vi "NI 9203_DOUBLETASK_AI.vi"(0 "MODULE NAME":string="CDR_AI", 1 "MODULE NAME 2":string="CDR_AI", 2 "sample mode":i32(ring)=10178 items=["Finite Samples"=10178, "Continuous Samples"=10123, "Hardware Timed Single Point"=12522], 3 "double task?":bool, 4 "rate":dbl=1000.0 format="%0.2f", 5 "error in":errorcluster) -> (14 "task out":refnum<k21>, 19 "error out":errorcluster)   [LabVIEW 2016]
uses:
  <vilib>/DAQmx/configure/timing.llb/DAQmx Timing (Sample Clock).vi
  <vilib>/DAQmx/create/channels.llb/DAQmx Create Channel (AI-Current-Basic).vi
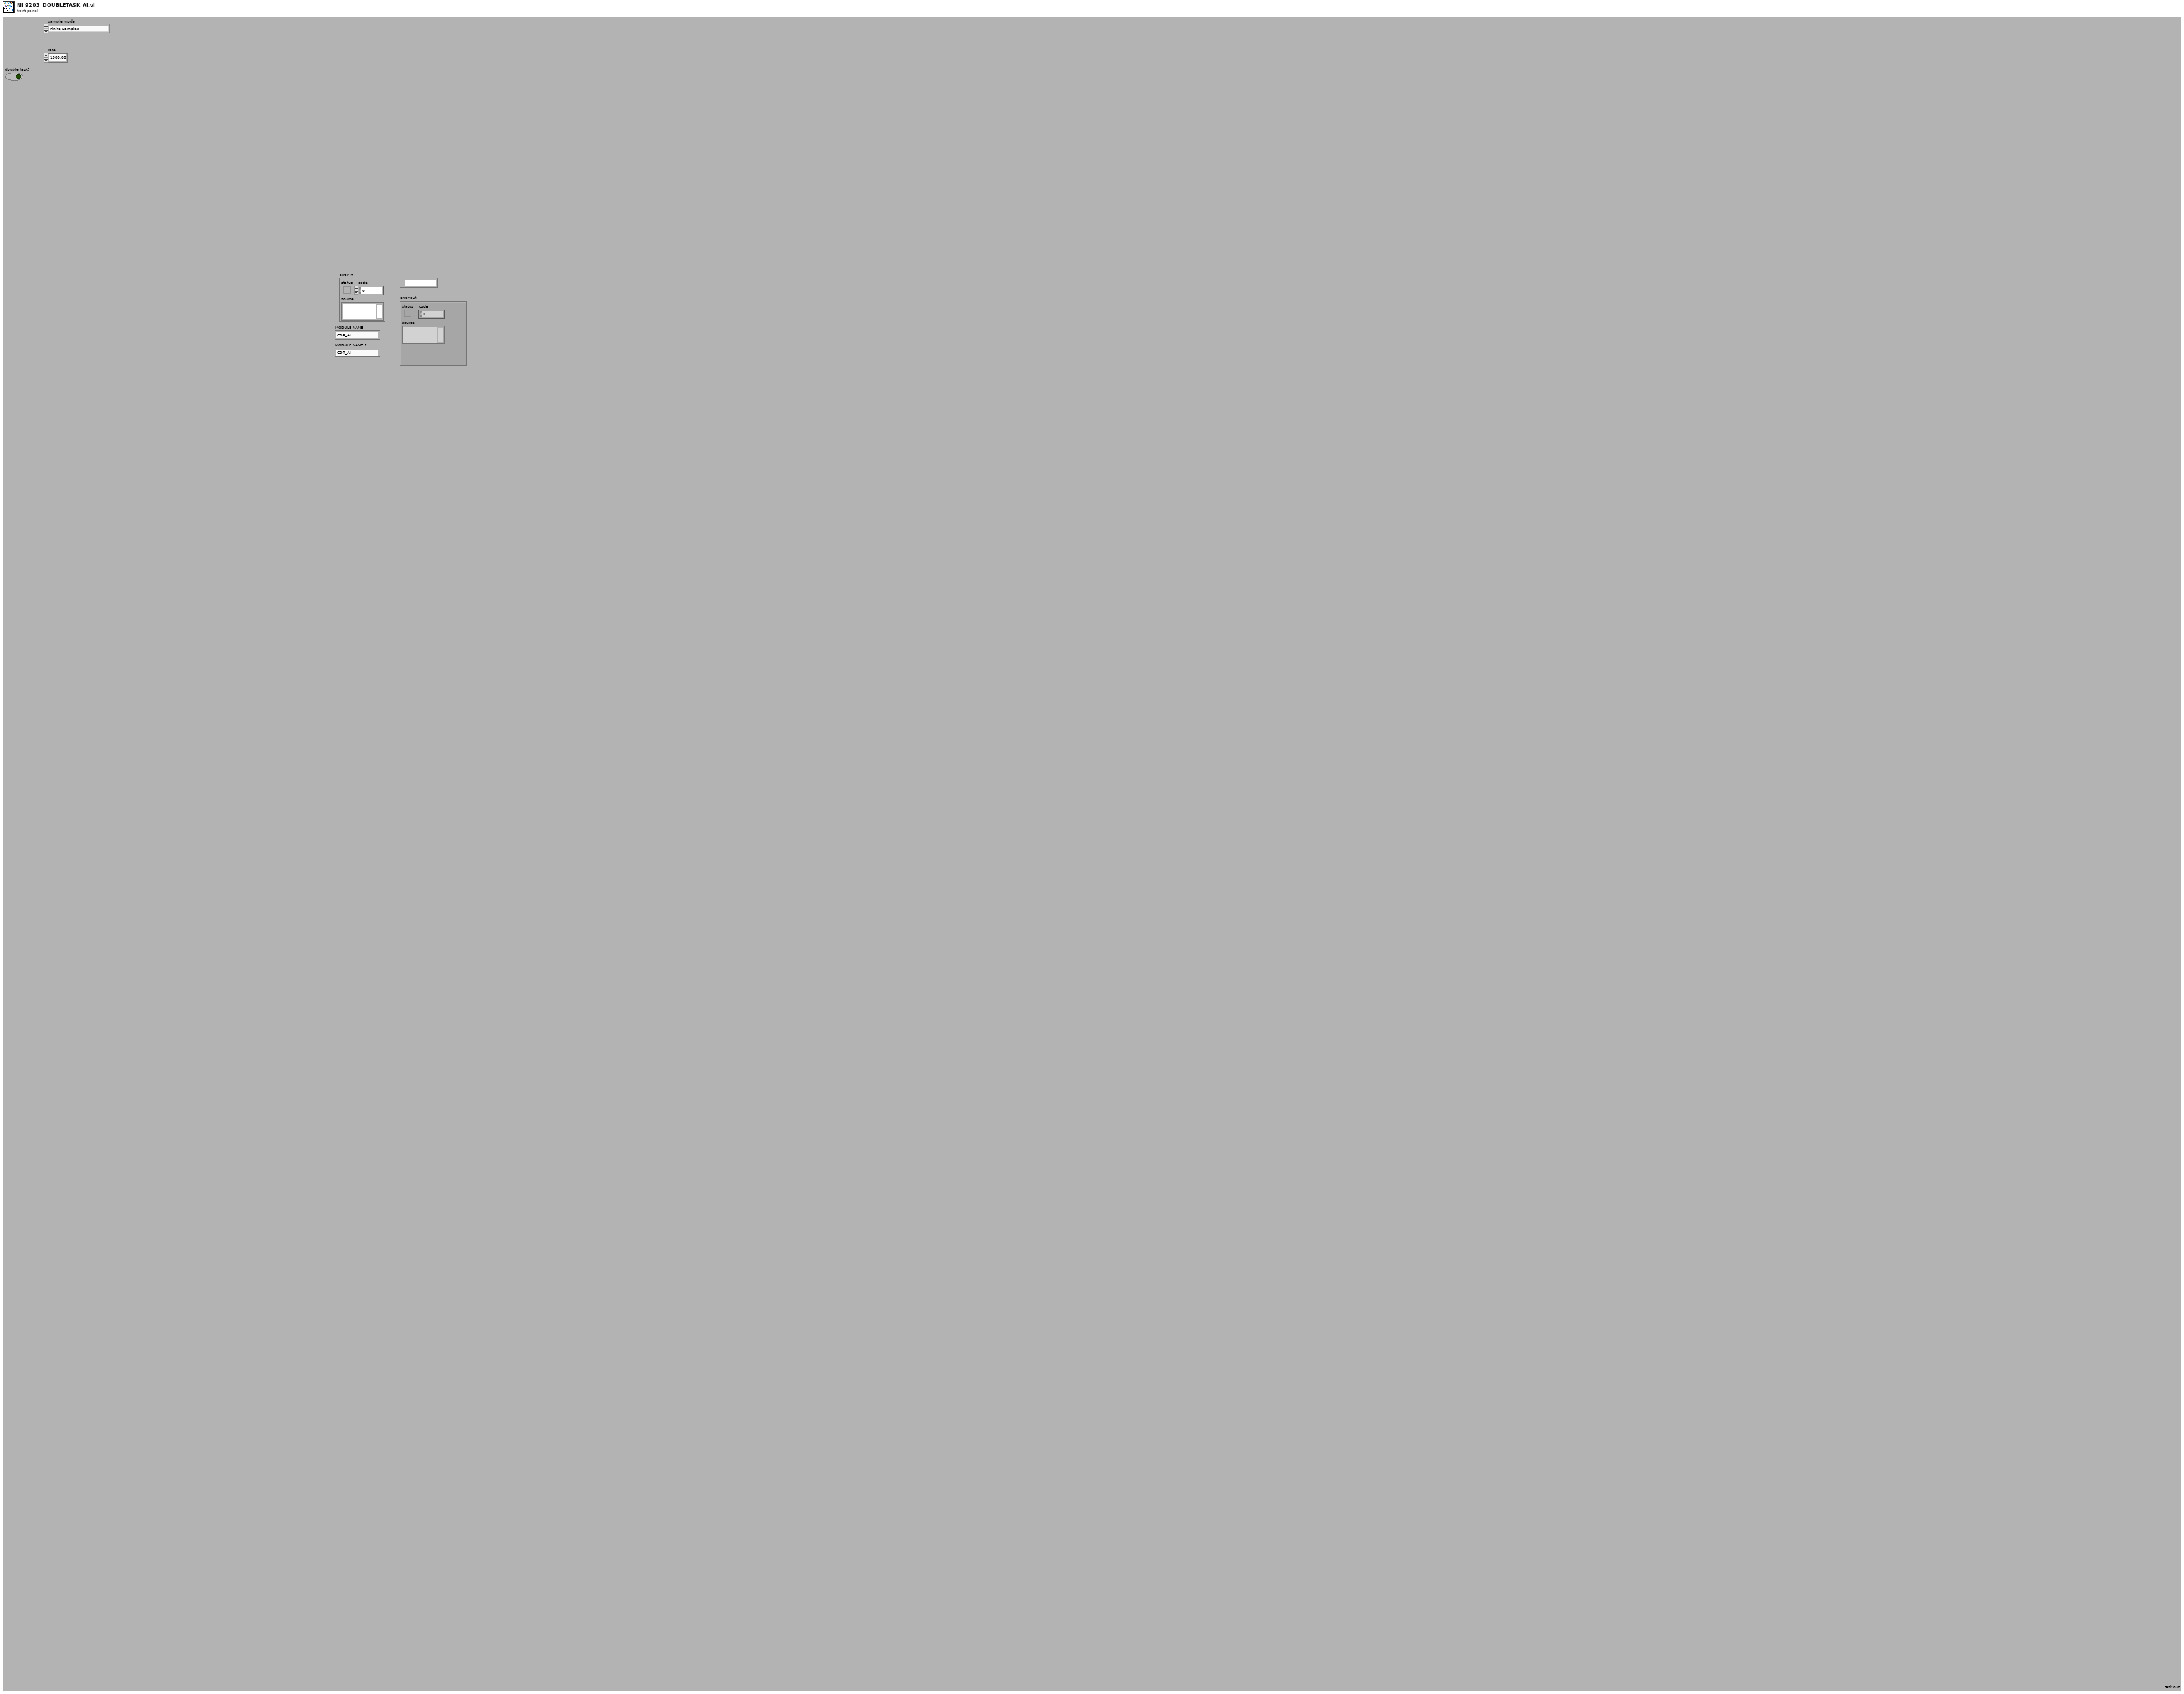
[diagram p1: front panel]
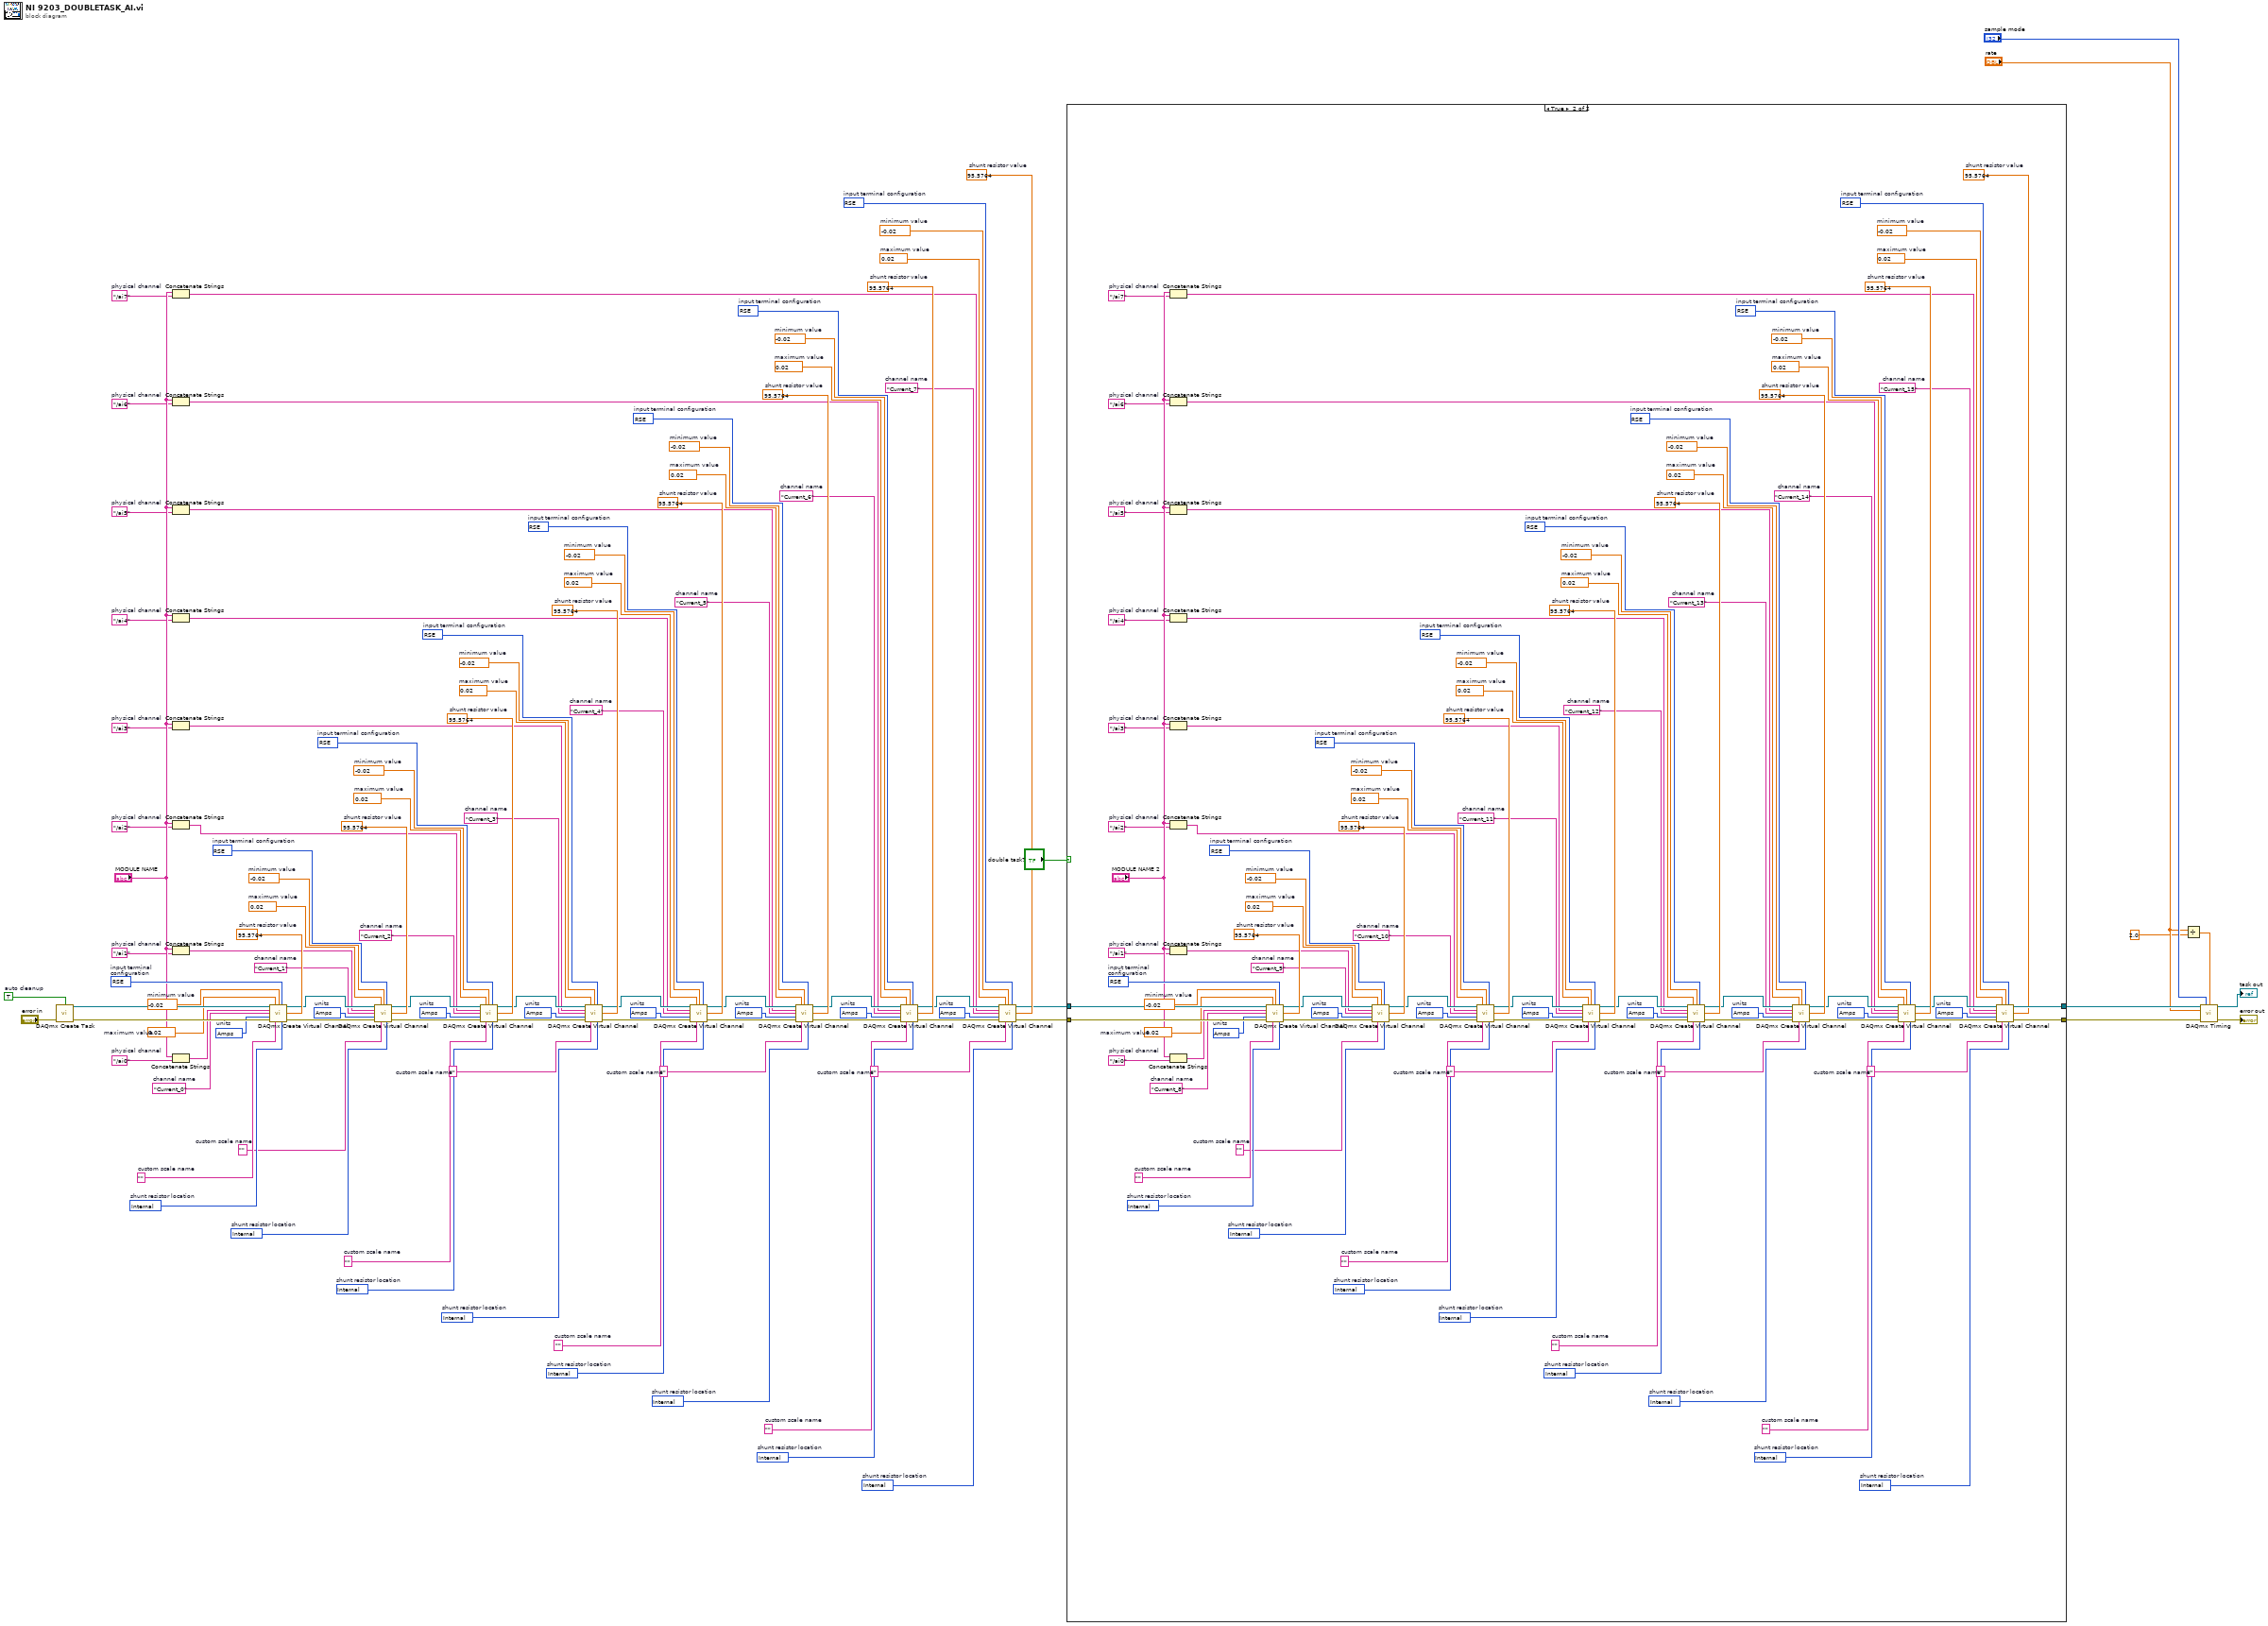
[diagram p0: block diagram]
diagram:
  w29 = 10083 items=["default"=-1, "RSE"=10083, "NRSE"=10078, "Differential"=10106, "Pseudodifferential"=12529]  # input terminal configuration
  w30 = 10342 items=["Amps"=10342, "From Custom Scale"=10065]  # units
  w31 = 95.5764  # shunt resistor value
  w32 = 10200 items=["Internal"=10200, "External"=10167]  # shunt resistor location
  w33 = "Current_7"  # channel name
  w34 = ""  # custom scale name
  w35 = -0.02  # minimum value
  w36 = 0.02  # maximum value
  w10 = "/ai7"  # physical channel
  w38 = 10083 items=["default"=-1, "RSE"=10083, "NRSE"=10078, "Differential"=10106, "Pseudodifferential"=12529]  # input terminal configuration
  w39 = 10342 items=["Amps"=10342, "From Custom Scale"=10065]  # units
  w40 = 95.5764  # shunt resistor value
  w41 = 10200 items=["Internal"=10200, "External"=10167]  # shunt resistor location
  w42 = "Current_6"  # channel name
  w44 = ""  # custom scale name
  w45 = -0.02  # minimum value
  w46 = 0.02  # maximum value
  w12 = "/ai6"  # physical channel
  w48 = 10083 items=["default"=-1, "RSE"=10083, "NRSE"=10078, "Differential"=10106, "Pseudodifferential"=12529]  # input terminal configuration
  w49 = 10342 items=["Amps"=10342, "From Custom Scale"=10065]  # units
  w50 = 95.5764  # shunt resistor value
  w51 = 10200 items=["Internal"=10200, "External"=10167]  # shunt resistor location
  w52 = "Current_5"  # channel name
  w54 = ""  # custom scale name
  w55 = -0.02  # minimum value
  w56 = 0.02  # maximum value
  w14 = "/ai5"  # physical channel
  w58 = 10083 items=["default"=-1, "RSE"=10083, "NRSE"=10078, "Differential"=10106, "Pseudodifferential"=12529]  # input terminal configuration
  w59 = 10342 items=["Amps"=10342, "From Custom Scale"=10065]  # units
  w60 = 95.5764  # shunt resistor value
  w61 = 10200 items=["Internal"=10200, "External"=10167]  # shunt resistor location
  w62 = "Current_4"  # channel name
  w64 = ""  # custom scale name
  w65 = -0.02  # minimum value
  w66 = 0.02  # maximum value
  w16 = "/ai4"  # physical channel
  w68 = 10083 items=["default"=-1, "RSE"=10083, "NRSE"=10078, "Differential"=10106, "Pseudodifferential"=12529]  # input terminal configuration
  w69 = 10342 items=["Amps"=10342, "From Custom Scale"=10065]  # units
  w70 = 95.5764  # shunt resistor value
  w71 = 10200 items=["Internal"=10200, "External"=10167]  # shunt resistor location
  w72 = "Current_3"  # channel name
  w74 = ""  # custom scale name
  w75 = -0.02  # minimum value
  w76 = 0.02  # maximum value
  w18 = "/ai3"  # physical channel
  w78 = 10083 items=["default"=-1, "RSE"=10083, "NRSE"=10078, "Differential"=10106, "Pseudodifferential"=12529]  # input terminal configuration
  w79 = 10342 items=["Amps"=10342, "From Custom Scale"=10065]  # units
  w80 = 95.5764  # shunt resistor value
  w81 = 10200 items=["Internal"=10200, "External"=10167]  # shunt resistor location
  w82 = "Current_2"  # channel name
  w84 = ""  # custom scale name
  w85 = -0.02  # minimum value
  w86 = 0.02  # maximum value
  w20 = "/ai2"  # physical channel
  w88 = 10083 items=["default"=-1, "RSE"=10083, "NRSE"=10078, "Differential"=10106, "Pseudodifferential"=12529]  # input terminal configuration
  w89 = 10342 items=["Amps"=10342, "From Custom Scale"=10065]  # units
  w90 = 95.5764  # shunt resistor value
  w91 = 10200 items=["Internal"=10200, "External"=10167]  # shunt resistor location
  w92 = "Current_1"  # channel name
  w94 = ""  # custom scale name
  w95 = -0.02  # minimum value
  w96 = 0.02  # maximum value
  w22 = "/ai1"  # physical channel
  w98 = 10083 items=["default"=-1, "RSE"=10083, "NRSE"=10078, "Differential"=10106, "Pseudodifferential"=12529]  # input terminal configuration
  w99 = 10342 items=["Amps"=10342, "From Custom Scale"=10065]  # units
  w100 = 95.5764  # shunt resistor value
  w101 = 10200 items=["Internal"=10200, "External"=10167]  # shunt resistor location
  w102 = "Current_0"  # channel name
  w104 = ""  # custom scale name
  w105 = -0.02  # minimum value
  w106 = 0.02  # maximum value
  w25 = "/ai0"  # physical channel
  w108 = TRUE  # auto cleanup
  n1 = call <vilib>:"DAQmx Create Task.vi"("auto cleanup"=w108, "error in"="error in") -> ("task out"=w107:refnum<k21>, "error out"=w109:errorcluster)  [unwired: 12 in]
  n2 = Concatenate Strings("MODULE NAME", w10) -> (w9:string)
  n3 = Concatenate Strings("MODULE NAME", w12) -> (w11:string)
  n4 = Concatenate Strings("MODULE NAME", w14) -> (w13:string)
  n5 = Concatenate Strings("MODULE NAME", w16) -> (w15:string)
  n6 = Concatenate Strings("MODULE NAME", w18) -> (w17:string)
  n7 = Concatenate Strings("MODULE NAME", w20) -> (w19:string)
  n8 = Concatenate Strings("MODULE NAME", w22) -> (w21:string)
  n9 = Concatenate Strings("MODULE NAME", w25) -> (w24:string)
  n10 = call-poly <vilib>:"DAQmx Create Virtual Channel.vi"("task in"=w107, "maximum value"=w106, "minimum value"=w105, "input terminal configuration"=w98, "physical channels"=w24, "name to assign"=w102, "external shunt resistor value"=w100, "units"=w99, "error in"=w109, "custom scale name"=w104, "shunt resistor location"=w101) -> ("task out"=w97:refnum<k21>, "error out"=w103:errorcluster)  [unwired: 3 in]
  n11 = call-poly <vilib>:"DAQmx Create Virtual Channel.vi"("task in"=w97, "maximum value"=w96, "minimum value"=w95, "input terminal configuration"=w88, "physical channels"=w21, "name to assign"=w92, "external shunt resistor value"=w90, "units"=w89, "error in"=w103, "custom scale name"=w94, "shunt resistor location"=w91) -> ("task out"=w87:refnum<k21>, "error out"=w93:errorcluster)  [unwired: 3 in]
  n12 = call-poly <vilib>:"DAQmx Create Virtual Channel.vi"("task in"=w87, "maximum value"=w86, "minimum value"=w85, "input terminal configuration"=w78, "physical channels"=w19, "name to assign"=w82, "external shunt resistor value"=w80, "units"=w79, "error in"=w93, "custom scale name"=w84, "shunt resistor location"=w81) -> ("task out"=w77:refnum<k21>, "error out"=w83:errorcluster)  [unwired: 3 in]
  n13 = call-poly <vilib>:"DAQmx Create Virtual Channel.vi"("task in"=w77, "maximum value"=w76, "minimum value"=w75, "input terminal configuration"=w68, "physical channels"=w17, "name to assign"=w72, "external shunt resistor value"=w70, "units"=w69, "error in"=w83, "custom scale name"=w74, "shunt resistor location"=w71) -> ("task out"=w67:refnum<k21>, "error out"=w73:errorcluster)  [unwired: 3 in]
  n14 = call-poly <vilib>:"DAQmx Create Virtual Channel.vi"("task in"=w67, "maximum value"=w66, "minimum value"=w65, "input terminal configuration"=w58, "physical channels"=w15, "name to assign"=w62, "external shunt resistor value"=w60, "units"=w59, "error in"=w73, "custom scale name"=w64, "shunt resistor location"=w61) -> ("task out"=w57:refnum<k21>, "error out"=w63:errorcluster)  [unwired: 3 in]
  n15 = call-poly <vilib>:"DAQmx Create Virtual Channel.vi"("task in"=w57, "maximum value"=w56, "minimum value"=w55, "input terminal configuration"=w48, "physical channels"=w13, "name to assign"=w52, "external shunt resistor value"=w50, "units"=w49, "error in"=w63, "custom scale name"=w54, "shunt resistor location"=w51) -> ("task out"=w47:refnum<k21>, "error out"=w53:errorcluster)  [unwired: 3 in]
  n16 = call-poly <vilib>:"DAQmx Create Virtual Channel.vi"("task in"=w47, "maximum value"=w46, "minimum value"=w45, "input terminal configuration"=w38, "physical channels"=w11, "name to assign"=w42, "external shunt resistor value"=w40, "units"=w39, "error in"=w53, "custom scale name"=w44, "shunt resistor location"=w41) -> ("task out"=w37:refnum<k21>, "error out"=w43:errorcluster)  [unwired: 3 in]
  n17 = call-poly <vilib>:"DAQmx Create Virtual Channel.vi"("task in"=w37, "maximum value"=w36, "minimum value"=w35, "input terminal configuration"=w29, "physical channels"=w9, "name to assign"=w33, "external shunt resistor value"=w31, "units"=w30, "error in"=w43, "custom scale name"=w34, "shunt resistor location"=w32) -> ("task out"=w7:refnum<k21>, "error out"=w8:errorcluster)  [unwired: 3 in]
  n18 = case shown="True" "double task?" {
    tunnel: w8 -> [w111 w211]
    tunnel: w7 -> [w112 w210]
    tunnel: [w112 w209] -> w6
    tunnel: [w111 w208] -> w5
    frame False {
    }
    frame True {
      w130 = 10083 items=["default"=-1, "RSE"=10083, "NRSE"=10078, "Differential"=10106, "Pseudodifferential"=12529]  # input terminal configuration
      w131 = 10342 items=["Amps"=10342, "From Custom Scale"=10065]  # units
      w132 = 95.5764  # shunt resistor value
      w133 = 10200 items=["Internal"=10200, "External"=10167]  # shunt resistor location
      w134 = "Current_15"  # channel name
      w135 = ""  # custom scale name
      w136 = -0.02  # minimum value
      w137 = 0.02  # maximum value
      w114 = "/ai7"  # physical channel
      w139 = 10083 items=["default"=-1, "RSE"=10083, "NRSE"=10078, "Differential"=10106, "Pseudodifferential"=12529]  # input terminal configuration
      w140 = 10342 items=["Amps"=10342, "From Custom Scale"=10065]  # units
      w141 = 95.5764  # shunt resistor value
      w142 = 10200 items=["Internal"=10200, "External"=10167]  # shunt resistor location
      w143 = "Current_14"  # channel name
      w145 = ""  # custom scale name
      w146 = -0.02  # minimum value
      w147 = 0.02  # maximum value
      w116 = "/ai6"  # physical channel
      w149 = 10083 items=["default"=-1, "RSE"=10083, "NRSE"=10078, "Differential"=10106, "Pseudodifferential"=12529]  # input terminal configuration
      w150 = 10342 items=["Amps"=10342, "From Custom Scale"=10065]  # units
      w151 = 95.5764  # shunt resistor value
      w152 = 10200 items=["Internal"=10200, "External"=10167]  # shunt resistor location
      w153 = "Current_13"  # channel name
      w155 = ""  # custom scale name
      w156 = -0.02  # minimum value
      w157 = 0.02  # maximum value
      w118 = "/ai5"  # physical channel
      w159 = 10083 items=["default"=-1, "RSE"=10083, "NRSE"=10078, "Differential"=10106, "Pseudodifferential"=12529]  # input terminal configuration
      w160 = 10342 items=["Amps"=10342, "From Custom Scale"=10065]  # units
      w161 = 95.5764  # shunt resistor value
      w162 = 10200 items=["Internal"=10200, "External"=10167]  # shunt resistor location
      w163 = "Current_12"  # channel name
      w165 = ""  # custom scale name
      w166 = -0.02  # minimum value
      w167 = 0.02  # maximum value
      w120 = "/ai4"  # physical channel
      w169 = 10083 items=["default"=-1, "RSE"=10083, "NRSE"=10078, "Differential"=10106, "Pseudodifferential"=12529]  # input terminal configuration
      w170 = 10342 items=["Amps"=10342, "From Custom Scale"=10065]  # units
      w171 = 95.5764  # shunt resistor value
      w172 = 10200 items=["Internal"=10200, "External"=10167]  # shunt resistor location
      w173 = "Current_11"  # channel name
      w175 = ""  # custom scale name
      w176 = -0.02  # minimum value
      w177 = 0.02  # maximum value
      w122 = "/ai3"  # physical channel
      w179 = 10083 items=["default"=-1, "RSE"=10083, "NRSE"=10078, "Differential"=10106, "Pseudodifferential"=12529]  # input terminal configuration
      w180 = 10342 items=["Amps"=10342, "From Custom Scale"=10065]  # units
      w181 = 95.5764  # shunt resistor value
      w182 = 10200 items=["Internal"=10200, "External"=10167]  # shunt resistor location
      w183 = "Current_10"  # channel name
      w185 = ""  # custom scale name
      w186 = -0.02  # minimum value
      w187 = 0.02  # maximum value
      w124 = "/ai2"  # physical channel
      w189 = 10083 items=["default"=-1, "RSE"=10083, "NRSE"=10078, "Differential"=10106, "Pseudodifferential"=12529]  # input terminal configuration
      w190 = 10342 items=["Amps"=10342, "From Custom Scale"=10065]  # units
      w191 = 95.5764  # shunt resistor value
      w192 = 10200 items=["Internal"=10200, "External"=10167]  # shunt resistor location
      w193 = "Current_9"  # channel name
      w195 = ""  # custom scale name
      w196 = -0.02  # minimum value
      w197 = 0.02  # maximum value
      w126 = "/ai1"  # physical channel
      w199 = 10083 items=["default"=-1, "RSE"=10083, "NRSE"=10078, "Differential"=10106, "Pseudodifferential"=12529]  # input terminal configuration
      w200 = 10342 items=["Amps"=10342, "From Custom Scale"=10065]  # units
      w201 = 95.5764  # shunt resistor value
      w202 = 10200 items=["Internal"=10200, "External"=10167]  # shunt resistor location
      w203 = "Current_8"  # channel name
      w205 = ""  # custom scale name
      w206 = -0.02  # minimum value
      w207 = 0.02  # maximum value
      w129 = "/ai0"  # physical channel
      n19 = Concatenate Strings("MODULE NAME 2", w114) -> (w113:string)
      n20 = Concatenate Strings("MODULE NAME 2", w116) -> (w115:string)
      n21 = Concatenate Strings("MODULE NAME 2", w118) -> (w117:string)
      n22 = Concatenate Strings("MODULE NAME 2", w120) -> (w119:string)
      n23 = Concatenate Strings("MODULE NAME 2", w122) -> (w121:string)
      n24 = Concatenate Strings("MODULE NAME 2", w124) -> (w123:string)
      n25 = Concatenate Strings("MODULE NAME 2", w126) -> (w125:string)
      n26 = Concatenate Strings("MODULE NAME 2", w129) -> (w128:string)
      n27 = call-poly <vilib>:"DAQmx Create Virtual Channel.vi"("task in"=w210, "maximum value"=w207, "minimum value"=w206, "input terminal configuration"=w199, "physical channels"=w128, "name to assign"=w203, "external shunt resistor value"=w201, "units"=w200, "error in"=w211, "custom scale name"=w205, "shunt resistor location"=w202) -> ("task out"=w198:refnum<k21>, "error out"=w204:errorcluster)  [unwired: 3 in]
      n28 = call-poly <vilib>:"DAQmx Create Virtual Channel.vi"("task in"=w198, "maximum value"=w197, "minimum value"=w196, "input terminal configuration"=w189, "physical channels"=w125, "name to assign"=w193, "external shunt resistor value"=w191, "units"=w190, "error in"=w204, "custom scale name"=w195, "shunt resistor location"=w192) -> ("task out"=w188:refnum<k21>, "error out"=w194:errorcluster)  [unwired: 3 in]
      n29 = call-poly <vilib>:"DAQmx Create Virtual Channel.vi"("task in"=w188, "maximum value"=w187, "minimum value"=w186, "input terminal configuration"=w179, "physical channels"=w123, "name to assign"=w183, "external shunt resistor value"=w181, "units"=w180, "error in"=w194, "custom scale name"=w185, "shunt resistor location"=w182) -> ("task out"=w178:refnum<k21>, "error out"=w184:errorcluster)  [unwired: 3 in]
      n30 = call-poly <vilib>:"DAQmx Create Virtual Channel.vi"("task in"=w178, "maximum value"=w177, "minimum value"=w176, "input terminal configuration"=w169, "physical channels"=w121, "name to assign"=w173, "external shunt resistor value"=w171, "units"=w170, "error in"=w184, "custom scale name"=w175, "shunt resistor location"=w172) -> ("task out"=w168:refnum<k21>, "error out"=w174:errorcluster)  [unwired: 3 in]
      n31 = call-poly <vilib>:"DAQmx Create Virtual Channel.vi"("task in"=w168, "maximum value"=w167, "minimum value"=w166, "input terminal configuration"=w159, "physical channels"=w119, "name to assign"=w163, "external shunt resistor value"=w161, "units"=w160, "error in"=w174, "custom scale name"=w165, "shunt resistor location"=w162) -> ("task out"=w158:refnum<k21>, "error out"=w164:errorcluster)  [unwired: 3 in]
      n32 = call-poly <vilib>:"DAQmx Create Virtual Channel.vi"("task in"=w158, "maximum value"=w157, "minimum value"=w156, "input terminal configuration"=w149, "physical channels"=w117, "name to assign"=w153, "external shunt resistor value"=w151, "units"=w150, "error in"=w164, "custom scale name"=w155, "shunt resistor location"=w152) -> ("task out"=w148:refnum<k21>, "error out"=w154:errorcluster)  [unwired: 3 in]
      n33 = call-poly <vilib>:"DAQmx Create Virtual Channel.vi"("task in"=w148, "maximum value"=w147, "minimum value"=w146, "input terminal configuration"=w139, "physical channels"=w115, "name to assign"=w143, "external shunt resistor value"=w141, "units"=w140, "error in"=w154, "custom scale name"=w145, "shunt resistor location"=w142) -> ("task out"=w138:refnum<k21>, "error out"=w144:errorcluster)  [unwired: 3 in]
      n34 = call-poly <vilib>:"DAQmx Create Virtual Channel.vi"("task in"=w138, "maximum value"=w137, "minimum value"=w136, "input terminal configuration"=w130, "physical channels"=w113, "name to assign"=w134, "external shunt resistor value"=w132, "units"=w131, "error in"=w144, "custom scale name"=w135, "shunt resistor location"=w133) -> ("task out"=w209:refnum<k21>, "error out"=w208:errorcluster)  [unwired: 3 in]
    }
  }
  n35 = Divide(x="rate", y=2.0) -> (x/y=w2:dbl)
  n36 = call-poly <vilib>:"DAQmx Timing.vi"("task/channels in"=w6, "sample mode"="sample mode", "samples per channel"=w2, "rate"="rate", "error in"=w5) -> ("task out"=→"task out":refnum<k21>, "error out"=→"error out":errorcluster)  [unwired: 9 in]
